vi "3_6var.vi"() -> ()   [LabVIEW 2022 SP3]
uses:
  5378e37b-4f60-4540-949a-2b5431a8859e.vi
  <vilib>/Comparison/Less/Less Functor/Less Functor.lvclass
panel:
  out "Output":string
  in  "stop":bool
  out "Array":string[](array[string])
  in  "Input":string
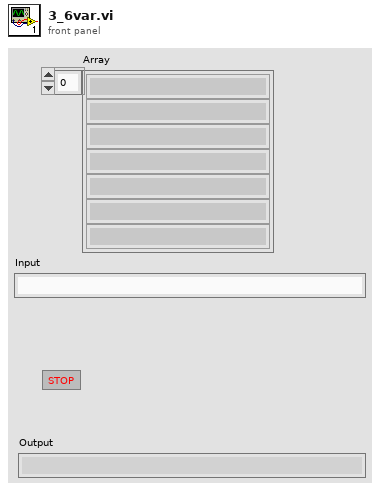
[diagram p1: front panel]
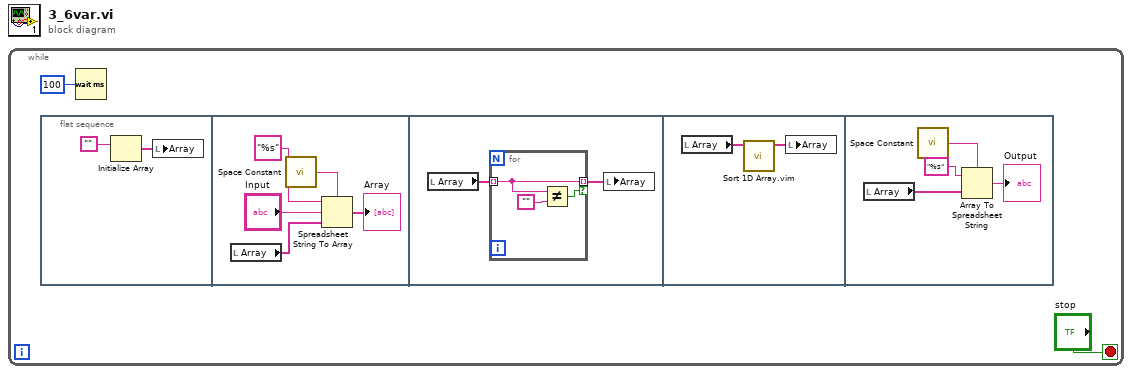
[diagram p0: block diagram]
diagram:
  n1 = while {
    stop <- "stop" stop-if-true
    n2 = flat-sequence {
      frame #0 {
        n3 = Initialize Array("") -> (w3:string[])  [unwired: 1 in]
        n4 = local write "Array"(w3) -> ()
      }
      frame #1 {
        n5 = local read "Array"() -> (w7:string[])
        n6 = call <vilib>:"Space Constant.vi"() -> ("String"=w9:string)
        n7 = Spreadsheet String To Array(delimiter (Tab)=w9, format string="%s", spreadsheet string="Input", array type (2D Dbl)=w7) -> (array=→"Array":string[])
      }
      frame #2 {
        n8 = local read "Array"() -> (w11:string[])
        n9 = for {
          tunnel: w11 -> [w13] mode=indexing
          tunnel: [w13] -> w10 mode=indexing if=w12
          n10 = Not Equal?(x=w13, y="") -> (x != y?=w12:bool)
        }
        n11 = local write "Array"(w10) -> ()
      }
      frame #3 {
        n12 = local read "Array"() -> (w16:string[])
        n13 = call "Sort 1D Array.vim"("unsorted array"=w16) -> ("sorted array"=w15:string[])  [unwired: 10 in]
        n14 = local write "Array"(w15) -> ()
      }
      frame #4 {
        n15 = local read "Array"() -> (w20:string[])
        n16 = call <vilib>:"Space Constant.vi"() -> ("String"=w19:string)
        n17 = Array To Spreadsheet String(delimiter (Tab)=w19, array=w20, 3:"%s") -> (spreadsheet string=→"Output":string)
      }
    }
    n18 = Wait (ms)(milliseconds to wait=100) -> ()  [unwired: 1 out]
  }
